vi "Read_all_waveforms.vi"(7 "Peak_data_in":cluster{dbl[], dbl[], dbl[], dbl[]}, 8 "Channel names":string[](array[string]), 9 "Group name":string, 10 "error in":errorcluster, 11 "tdms file in":refnum<k34>) -> (0 "Waveforms":waveform(dbl)[](array[waveform]), 1 "Spectrum":T1(array[cluster]), 2 "error out":errorcluster, 3 "tdms file out":refnum<k34>, 5 "Peak_data_out":cluster{dbl[], dbl[], dbl[], dbl[]})   [LabVIEW 2019]
uses:
  SiPM_Tests_Global_Var.vi
  Agilent_lib/Agilent 2000 3000 X-Series.lvlib
  <vilib>/Analysis/NI_AALPro.lvlib
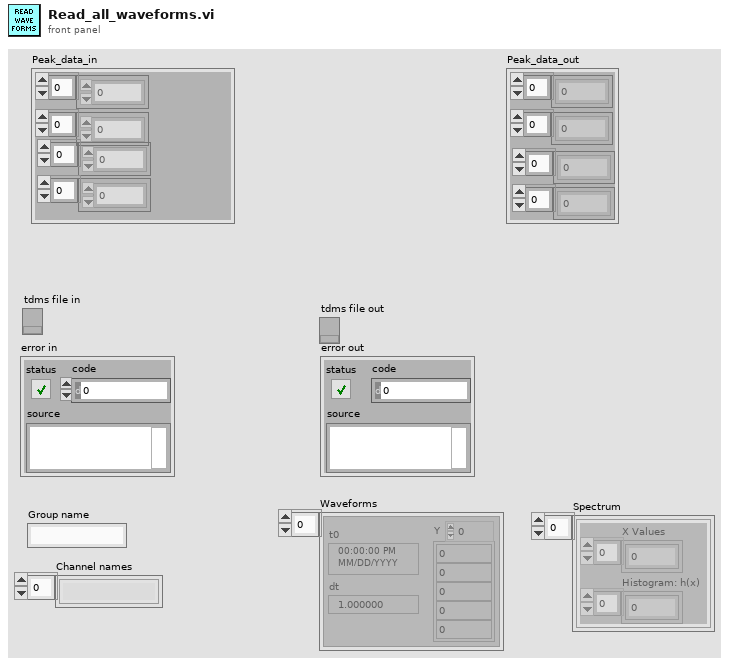
[diagram p1: front panel]
types:
  T1 = cluster{"X Values":dbl[], "Histogram: h(x)":i32[]}[]
  T2 = cluster{"X Values":dbl[], "Histogram: h(x)":i32[]}
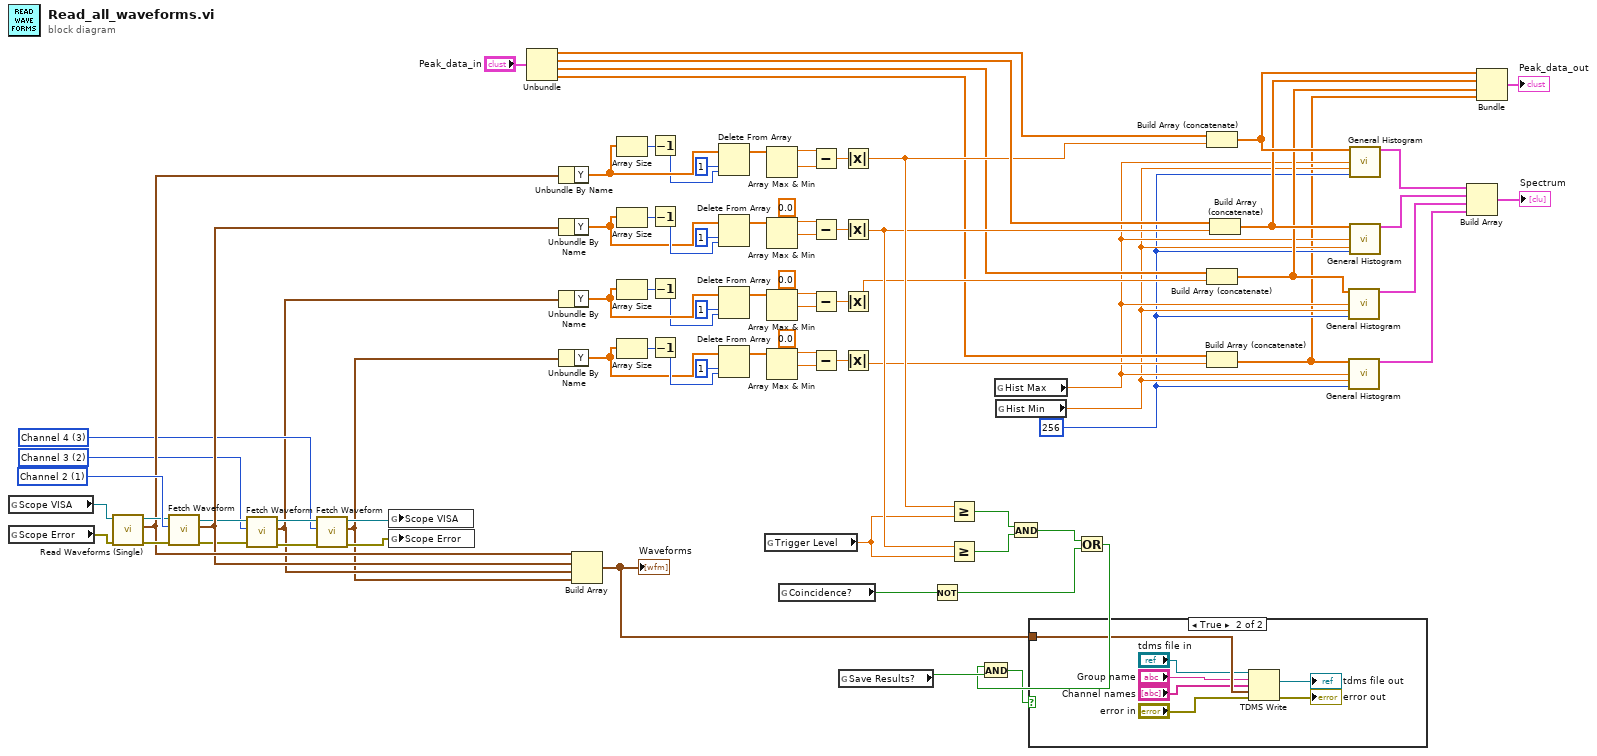
[diagram p0: block diagram]
diagram:
  (unwired) 0.0 ("y")
  (unwired) 0.0 ("y")
  w33 = 3 items=["Channel 1"=0, "Channel 2"=1, "Channel 3"=2, "Channel 4"=3, "Waveform Memory 1"=5, "Waveform Memory 2"=6, "Serial Bus 1"=7, "Serial Bus 2"=8, "Digital Bus Low"=9, "Digital Bus High "=10, "Digital Bus 1"=11, "Digital Bus 2"=12, "Function 1"=32, "Function 2"=33, "Function 3"=34, "Function 4"=35, "Math 1"=36, "Math 2"=37, "Math 3"=38, "Math 4"=39] ("Source Channel (0: Channel 1)")
  w36 = 2 items=["Channel 1"=0, "Channel 2"=1, "Channel 3"=2, "Channel 4"=3, "Waveform Memory 1"=5, "Waveform Memory 2"=6, "Serial Bus 1"=7, "Serial Bus 2"=8, "Digital Bus Low"=9, "Digital Bus High "=10, "Digital Bus 1"=11, "Digital Bus 2"=12, "Function 1"=32, "Function 2"=33, "Function 3"=34, "Function 4"=35, "Math 1"=36, "Math 2"=37, "Math 3"=38, "Math 4"=39] ("Source Channel (0: Channel 1)")
  (unwired) 0.0 ("y")
  w3 = 256 ("# bins")
  w81 = 1 items=["Channel 1"=0, "Channel 2"=1, "Channel 3"=2, "Channel 4"=3, "Waveform Memory 1"=5, "Waveform Memory 2"=6, "Serial Bus 1"=7, "Serial Bus 2"=8, "Digital Bus Low"=9, "Digital Bus High "=10, "Digital Bus 1"=11, "Digital Bus 2"=12, "Function 1"=32, "Function 2"=33, "Function 3"=34, "Function 4"=35, "Math 1"=36, "Math 2"=37, "Math 3"=38, "Math 4"=39] ("Source Channel (0: Channel 1)")
  n1 = global read "SiPM_Tests_Global_Var.vi" "Scope VISA"() -> (w76:refnum<visa-resource-name>)
  n2 = global read "SiPM_Tests_Global_Var.vi" "Scope Error"() -> (w77:errorcluster)
  n3 = call "Read Waveforms (Single).vi"("error in (no error)"=w77, "VISA resource name"=w76) -> ("error out"=w79:errorcluster, "Waveform Data"=w75:waveform(dbl), "VISA resource name out"=w78:refnum<visa-resource-name>)  [unwired: 7 in]
  n4 = call "Fetch Waveform.vi"("error in (no error)"=w79, "Source Channel (0: Channel 1)"=w81, "VISA resource name"=w78) -> ("error out"=w37:errorcluster, "Waveform Data"=w74:waveform(dbl), "VISA resource name out"=w38:refnum<visa-resource-name>)  [unwired: 2 in, 4 out]
  n5 = call "Fetch Waveform.vi"("error in (no error)"=w37, "Source Channel (0: Channel 1)"=w36, "VISA resource name"=w38) -> ("error out"=w35:errorcluster, "Waveform Data"=w24:waveform(dbl), "VISA resource name out"=w34:refnum<visa-resource-name>)  [unwired: 2 in, 4 out]
  n6 = call "Fetch Waveform.vi"("error in (no error)"=w35, "Source Channel (0: Channel 1)"=w33, "VISA resource name"=w34) -> ("error out"=w22:errorcluster, "Waveform Data"=w13:waveform(dbl), "VISA resource name out"=w23:refnum<visa-resource-name>)  [unwired: 2 in, 4 out]
  n7 = global write "SiPM_Tests_Global_Var.vi" "Scope VISA"(w23) -> ()
  n8 = global write "SiPM_Tests_Global_Var.vi" "Scope Error"(w22) -> ()
  n9 = Unbundle("Peak_data_in") -> (w56:dbl[], w55:dbl[], w8:dbl[], w7:dbl[])
  n10 = Unbundle By Name(w75) -> ("Y"=w67:dbl[])
  n11 = Unbundle By Name(w74) -> ("Y"=w58:dbl[])
  n12 = Unbundle By Name(w24) -> ("Y"=w31:dbl[])
  n13 = Unbundle By Name(w13) -> ("Y"=w15:dbl[])
  n14 = Build Array(w75, w74, w24, w13) -> (w80:waveform(dbl)[])
  "Waveforms" <- w80
  n15 = Array Size(array=w67) -> (size(s)=w66:i32)
  n16 = Array Size(array=w58) -> (size(s)=w63:i32)
  n17 = Array Size(array=w31) -> (size(s)=w26:i32)
  n18 = Array Size(array=w15) -> (size(s)=w20:i32)
  n19 = Decrement(x=w66) -> (x-1=w65:i32)
  n20 = Decrement(x=w63) -> (x-1=w64:i32)
  n21 = Decrement(x=w26) -> (x-1=w25:i32)
  n22 = Decrement(x=w20) -> (x-1=w21:i32)
  n23 = Delete From Array(array=w67, length=1, index=w65) -> (array with subset deleted=w69:dbl[])  [unwired: 1 out]
  n24 = Delete From Array(array=w58, length=1, index=w64) -> (array with subset deleted=w61:dbl[])  [unwired: 1 out]
  n25 = Delete From Array(array=w31, length=1, index=w25) -> (array with subset deleted=w28:dbl[])  [unwired: 1 out]
  n26 = Delete From Array(array=w15, length=1, index=w21) -> (array with subset deleted=w18:dbl[])  [unwired: 1 out]
  n27 = global read "SiPM_Tests_Global_Var.vi" "Trigger Level"() -> (w49:dbl)
  n28 = Array Max & Min(array=w69) -> (max value=w73:dbl, min value=w40:dbl)  [unwired: 2 out]
  n29 = Array Max & Min(array=w61) -> (max value=w59:dbl, min value=w39:dbl)  [unwired: 2 out]
  n30 = Array Max & Min(array=w28) -> (max value=w30:dbl, min value=w32:dbl)  [unwired: 2 out]
  n31 = Array Max & Min(array=w18) -> (max value=w16:dbl, min value=w14:dbl)  [unwired: 2 out]
  n32 = global read "SiPM_Tests_Global_Var.vi" "Coincidence?"() -> (w45:bool)
  n33 = Subtract(x=w73, y=w40) -> (x-y=w72:dbl)
  n34 = Subtract(x=w59, y=w39) -> (x-y=w60:dbl)
  n35 = Subtract(x=w30, y=w32) -> (x-y=w29:dbl)
  n36 = Subtract(x=w16, y=w14) -> (x-y=w17:dbl)
  n37 = global read "SiPM_Tests_Global_Var.vi" "Save Results?"() -> (w43:bool)
  n38 = Absolute Value(x=w72) -> (abs(x)=w51:dbl)
  n39 = Absolute Value(x=w60) -> (abs(x)=w50:dbl)
  n40 = Absolute Value(x=w29) -> (abs(x)=w10:dbl)
  n41 = Absolute Value(x=w17) -> (abs(x)=w6:dbl)
  n42 = Not(x=w45) -> (.not. x?=w44:bool)
  n43 = Greater Or Equal?(x=w51, y=w49) -> (x >= y?=w48:bool)
  n44 = Greater Or Equal?(x=w50, y=w49) -> (x >= y?=w47:bool)
  n45 = global read "SiPM_Tests_Global_Var.vi" "Hist Max"() -> (w5:dbl)
  n46 = global read "SiPM_Tests_Global_Var.vi" "Hist Min"() -> (w4:dbl)
  n47 = And(x=w48, y=w47) -> (x .and. y?=w46:bool)
  n48 = Or(x=w46, y=w44) -> (x .or. y?=w42:bool)
  n49 = And(x=w42, y=w43) -> (x .and. y?=w41:bool)
  n50 = case shown="True" w41 {
    tunnel: w80 -> [_ w88]
    frame False {
    }
    frame True {
      n51 = TDMS Write(0:"tdms file in", 5:"Group name", 7:"Channel names", 9:w88, 11:"error in") -> (4:→"tdms file out":refnum<k34>, 15:→"error out":errorcluster)  [unwired: 1 in, 2 out]
    }
  }
  n52 = Build Array (concatenate)(w56, w51) -> (w54:dbl[])
  n53 = Build Array (concatenate)(w8, w10) -> (w9:dbl[])
  n54 = Build Array (concatenate)(w7, w6) -> (w2:dbl[])
  n55 = Build Array (concatenate)(w55, w50) -> (w53:dbl[])
  n56 = call <vilib>:"General Histogram.vi"("X"=w9, "max"=w5, "min"=w4, "# bins"=w3) -> ("Histogram Graph"=w12:T2)  [unwired: 7 in, 4 out]
  n57 = call <vilib>:"General Histogram.vi"("X"=w2, "max"=w5, "min"=w4, "# bins"=w3) -> ("Histogram Graph"=w11:T2)  [unwired: 7 in, 4 out]
  n58 = call <vilib>:"General Histogram.vi"("X"=w54, "max"=w5, "min"=w4, "# bins"=w3) -> ("Histogram Graph"=w71:T2)  [unwired: 7 in, 4 out]
  n59 = call <vilib>:"General Histogram.vi"("X"=w53, "max"=w5, "min"=w4, "# bins"=w3) -> ("Histogram Graph"=w57:T2)  [unwired: 7 in, 4 out]
  n60 = Build Array(w71, w57, w12, w11) -> (→"Spectrum":T1)
  n61 = Bundle(w54, w53, w9, w2) -> (→"Peak_data_out":cluster{dbl[], dbl[], dbl[], dbl[]})  [unwired: 1 in]
